vi "Get VI Inputs and Outputs [Variant].vi"(8 "error in (no error)":errorcluster, 11 "VI Refnum":refnum<vi>) -> (0 "error out":errorcluster, 1 "VI Name":string, 2 "Outputs[]":cluster{"Name":string, "Value":variant}[](array[cluster]), 3 "Inputs[]":cluster{"Name":string, "Value":variant}[](array[cluster]))   [LabVIEW 2016, in "SLL Application.lvlib"]
uses:
  SLL Application.lvlib
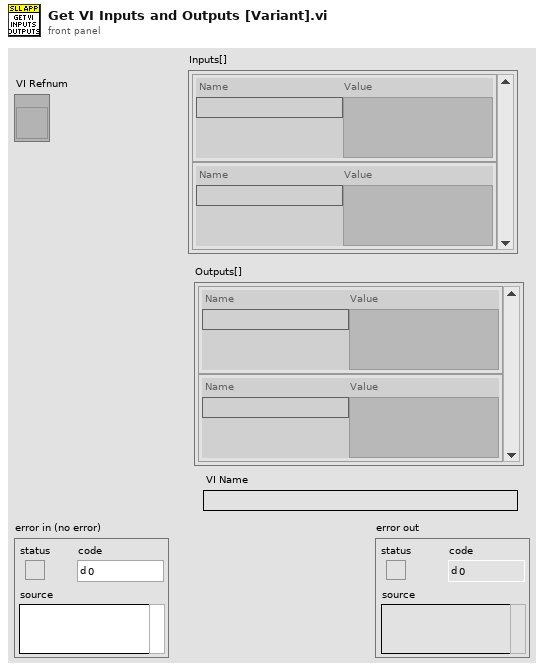
[diagram p1: front panel]
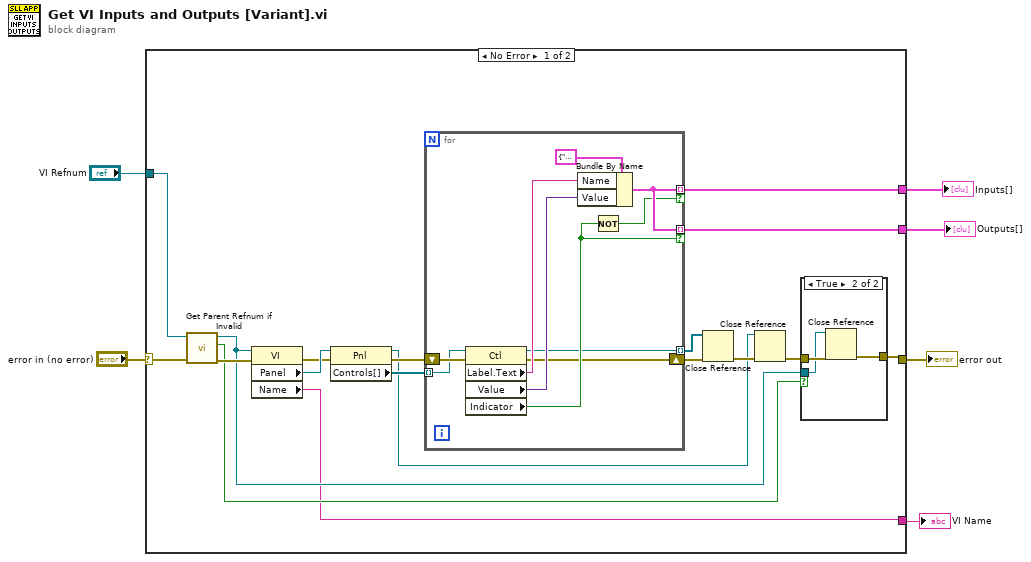
[diagram p0: block diagram]
diagram:
  n1 = case shown="No Error" "error in (no error)" {
    selector: "error in (no error)" -> [w14 w39]
    tunnel: [w8 w39] -> w5
    tunnel: "VI Refnum" -> [w12 _]
    tunnel: [w20 _] -> w3
    tunnel: [w19 _] -> w2
    tunnel: [w7 _] -> w1
    frame No Error {
      n2 = call "Get Parent Refnum if Invalid.vi"("error in (no error)"=w14, "VI Refnum In"=w12) -> ("error out"=w13:errorcluster, "Invalid?"=w10:bool, "VI Refnum Out"=w9:refnum<vi>)  [unwired: 7 in]
      n3 = property class="VI"(reference=w9, error in=w13) -> (error out=w23:errorcluster, "Panel"=w24:refnum<vi>, "Name"=w7:string)  [unwired: 1 out]
      n4 = property class="Pnl"(reference=w24, error in=w23) -> (reference out=w15:refnum<vi>, error out=w22:errorcluster, "Controls[]"=w21:refnum<vi>[])
      n5 = for {
        tunnel: w21 -> [w37] mode=indexing
        tunnel: [w33] -> w20 mode=indexing if=w31
        tunnel: [w33] -> w19 mode=indexing if=w32
        shift-right: [w30] -> w18
        shift-left: w22 -> [w38]
        tunnel: [w29] -> w17 mode=indexing
        n6 = property class="Ctl"(reference=w37, error in=w38) -> (reference out=w29:refnum<vi>, error out=w30:errorcluster, "Label.Text"=w35:string, "Value"=w34:variant, "Indicator"=w32:bool)
        n7 = Bundle By Name(cluster=cluster{"Name":string, "Value":variant} {"Name"="", "Value"=variant} ("System Cluster"), "Name"=w35, "Value"=w34) -> (w33:cluster{"Name":string, "Value":variant})
        n8 = Not(x=w32) -> (.not. x?=w31:bool)
      }
      n9 = Close Reference(reference=w17, error in (no error)=w18) -> (error out=w16:errorcluster)
      n10 = Close Reference(reference=w15, error in (no error)=w16) -> (error out=w11:errorcluster)
      n11 = case shown="True" w10 {
        tunnel: w11 -> [w25 w28]
        tunnel: w9 -> [_ w26]
        tunnel: [w25 w27] -> w8
        frame False {
        }
        frame True {
          n12 = Close Reference(reference=w26, error in (no error)=w28) -> (error out=w27:errorcluster)
        }
      }
    }
    frame Error {
    }
  }
  "error out" <- w5
  "Inputs[]" <- w3
  "Outputs[]" <- w2
  "VI Name" <- w1
